vi "PH_BL-Master.get Status of Status Service Subscriber by Name.vi"(0 "i ref in":refnum<vi>, 2 "Status Subscriber Instance":string="N/A", 5 "error in (no error)":errorcluster) -> (14 "i ref out":refnum<vi>, 16 "Status Subscriber Information":T1, 19 "error out":errorcluster)   [LabVIEW 2014, in "PH_BL-Master.lvlib"]
doc: "This VI gets the status of the selected Subscriber."
uses:
  PH_BL-Master.lvlib
  PH_BL-Master.Status Subscriber Information.ctl
  PH_BL-Master.Attribute Set.ctl
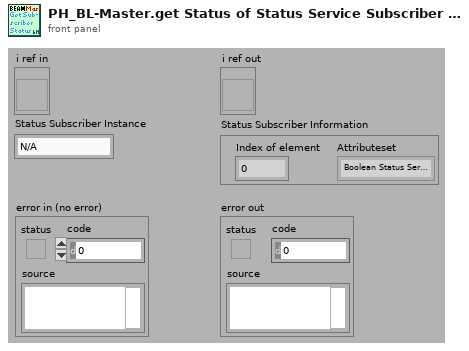
[diagram p1: front panel]
types:
  T1 = typedef "PH_BL-Master.lvlib/PH_BL-Master.Status Subscriber Information.ctl" = cluster{"Index of element":i32, "Attributeset":T2}
  T2 = typedef "PH_BL-Master.lvlib/PH_BL-Master.Attribute Set.ctl" = enum16{"Boolean Status Service Subscriber", "Picture Status Service Subscriber"}
  T3 = typedef "PH_BL-Master.lvlib/PH_BL-Master.i attribute.ctl" = cluster{"Remote controlled":bool, "Boolean Condition Service Subscriber":refnum<vi>[], "Picture Condition Service Subscriber":refnum<vi>[], "R2S":cluster{"GUI Ref":refnum<vi>, "State":bool}, "Vacua":cluster{"GUI Ref":refnum<vi>, "Limit":dbl, "Curr Value":dbl, "in range":bool}[], "O2 Inspection":cluster{"GUI Ref":refnum<vi>, "Concentration":dbl, "State":T4}[], "Boolean Status Service Subscriber":cluster{"GUI Ref":refnum<vi>, "Status":T4, "no Link?":bool, "Status Subscriber Class":T5}[], "Picture Status Service Subscriber":cluster{"GUI Ref":refnum<vi>, "Status":T4, "no Link?":bool, "Status Subscriber Class":T5}[], "6P 4Q Service Subscriber":cluster{"GUI Ref":refnum<vi>, "Selector":T6, "no Link?":bool}[], "Index of latest 6P 4Q changing Instance":i32, "Index of latest Picture Status changing Instance":i32, "Index of latest Boolean Status changing Instance":i32, "Vision ID on same Node":string, "Start Phase over?":bool, "GUI Ref Delete":refnum<vi>}
  T4 = typedef "PH_StatusHandler.lvlib/PH_StatusHandler.Status.ctl" = i16
  T5 = typedef "PH_BL-Master.lvlib/PH_BL-Master.Status Subscriber Class.ctl" = enum16{"unknown", "Switch", "BB", "6P Switch", "Switch GUI", "Switch and 6P State", "Force Sensor"}
  T6 = typedef "PH_4_Pos_Selector.lvlib/PH_4_Pos_Selector.Position Selector.ctl" = u16
  T7 = cluster{"GUI Ref":refnum<vi>, "Status":T4, "no Link?":bool, "Status Subscriber Class":T5}[]
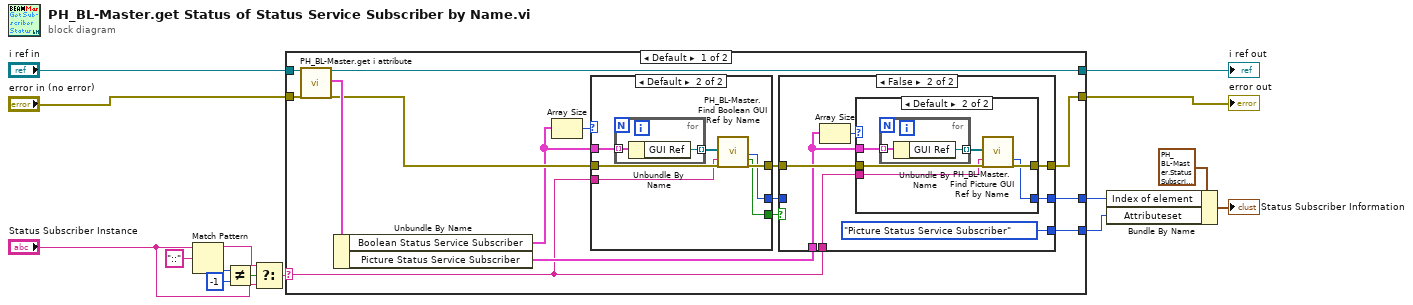
[diagram p0: block diagram]
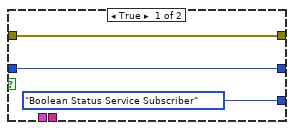
[diagram p2: hidden frame]
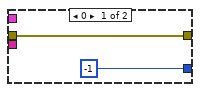
[diagram p3: hidden frame]
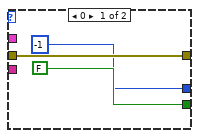
[diagram p4: hidden frame]
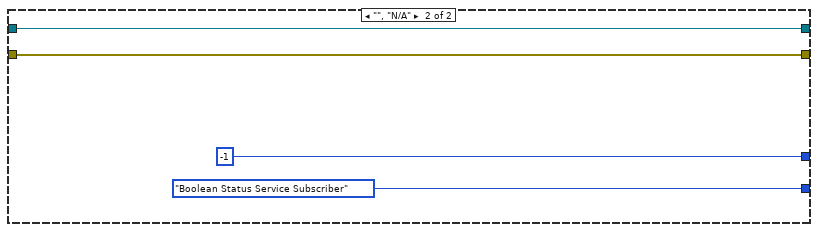
[diagram p5: hidden frame]
diagram:
  n1 = Match Pattern(string="Status Subscriber Instance", regular expression="::") -> (before substring=w5:string, offset past match=w10:i32)  [unwired: 1 in, 2 out]
  n2 = Not Equal?(x=w10, y=-1) -> (x != y?=w8:bool)
  n3 = Select(t=w5, s=w8, f="Status Subscriber Instance") -> (s? t:f=w6:string)
  n4 = case shown="Default" w6 {
    selector: w6 -> [w20 _]
    tunnel: "error in (no error)" -> [w29 w65]
    tunnel: "i ref in" -> [w28 w66]
    tunnel: [w27 w66] -> w12
    tunnel: [w22 w65] -> w13
    tunnel: [w17 -1 ("index of element")] -> w2
    tunnel: [w16 PH_BL-Master.Attribute_Set."Boolean Status Service Subscriber" ("Attributeset")] -> w1
    frame Default {
      n5 = call "PH_BL-Master.get i attribute.vi"("i ref in"=w28, "error in (no error)"=w29) -> ("i ref out"=w27:refnum<vi>, "i attribute"=w30:T3, "error out"=w25:errorcluster)  [unwired: 15 in]
      n6 = Unbundle By Name(w30) -> ("Boolean Status Service Subscriber"=w24:T7, "Picture Status Service Subscriber"=w21:T7)
      n7 = Array Size(array=w24) -> (size(s)=w26:i32)
      n8 = case shown="Default" w26 {
        tunnel: w24 -> [_ w57]
        tunnel: w20 -> [_ w58]
        tunnel: [w53 w56] -> w23
        tunnel: w25 -> [w53 w59]
        tunnel: [FALSE ("Ref found?") w55] -> w19
        tunnel: [-1 ("index of element") w54] -> w18
        frame 0 {
        }
        frame Default {
          n9 = for {
            tunnel: w57 -> [w62] mode=indexing
            tunnel: [w61] -> w60 mode=indexing
            n10 = Unbundle By Name(w62) -> ("GUI Ref"=w61:refnum<vi>)
          }
          n11 = call "PH_BL-Master.Find Boolean GUI Ref by Name.vi"("Boolean Ref Array"=w60, "Label"=w58, "error in (no error)"=w59) -> ("index of element"=w54:i32, "Ref found?"=w55:bool, "error out"=w56:errorcluster)  [unwired: 13 in, 1 out]
        }
      }
      n12 = case shown="False" w19 {
        tunnel: w23 -> [w33 w40]
        tunnel: [w33 w39] -> w22
        tunnel: w21 -> [_ w37]
        tunnel: w20 -> [_ w36]
        tunnel: w18 -> [w32 _]
        tunnel: [w32 w35] -> w17
        tunnel: [PH_BL-Master.Attribute_Set."Boolean Status Service Subscriber" ("Attributeset") PH_BL-Master.Attribute_Set."Picture Status Service Subscriber" ("Attributeset")] -> w16
        frame True {
        }
        frame False {
          n13 = Array Size(array=w37) -> (size(s)=w38:i32)
          n14 = case shown="Default" w38 {
            tunnel: w37 -> [_ w46]
            tunnel: w36 -> [_ w43]
            tunnel: [w42 w45] -> w39
            tunnel: w40 -> [w42 w47]
            tunnel: [-1 ("index of element") w44] -> w35
            frame 0 {
            }
            frame Default {
              n15 = for {
                tunnel: w46 -> [w50] mode=indexing
                tunnel: [w49] -> w48 mode=indexing
                n16 = Unbundle By Name(w50) -> ("GUI Ref"=w49:refnum<vi>)
              }
              n17 = call "PH_BL-Master.Find Picture GUI Ref by Name.vi"("Pic Ref Array"=w48, "Label"=w43, "error in"=w47) -> ("index of element"=w44:i32, "error out"=w45:errorcluster)  [unwired: 13 in, 2 out]
            }
          }
        }
      }
    }
    frame "", "N/A" {
    }
  }
  "i ref out" <- w12
  "error out" <- w13
  n18 = Bundle By Name(cluster=T1 {"Index of element"=0, "Attributeset"=enum."Boolean Status Service Subscriber"} ("Status Subscriber Information"), "Index of element"=w2, "Attributeset"=w1) -> (→"Status Subscriber Information":T1)
